vi "快捷菜单激活(表格).vi"(11 "菜单引用":refnum<k9>) -> ()   [LabVIEW 2021]
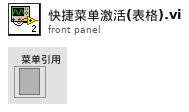
[diagram p1: front panel]
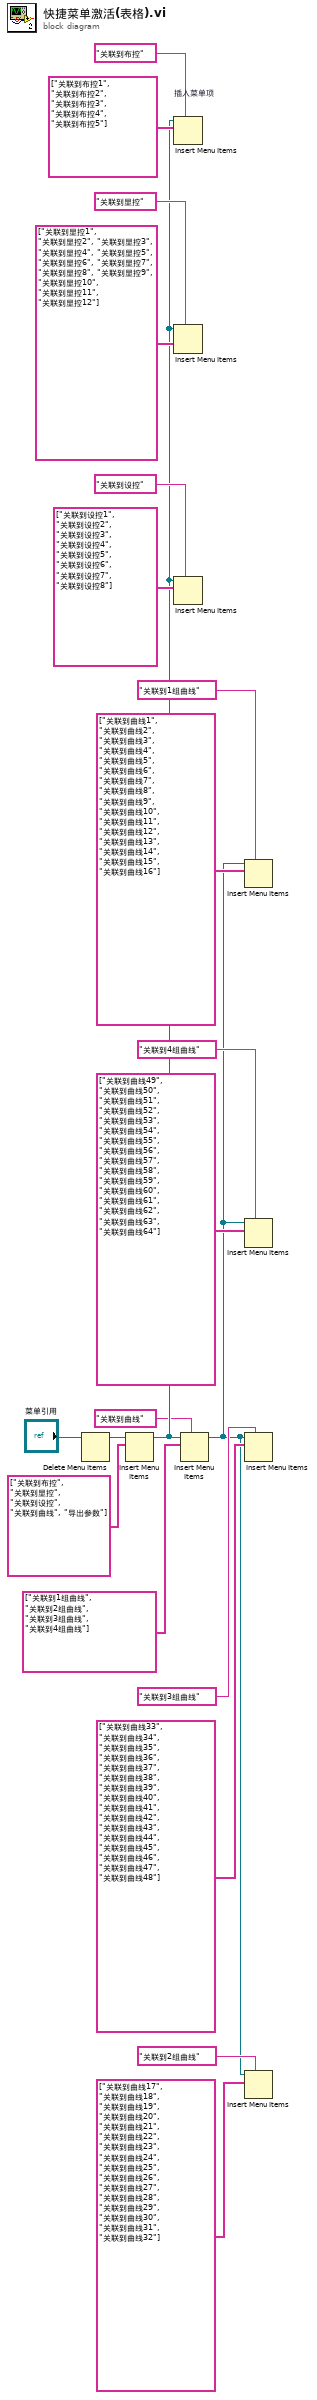
[diagram p0: block diagram]
diagram:
  n1 = Delete Menu Items(9:"菜单引用") -> (3:w21:refnum<k9>)  [unwired: 3 in, 1 out]
  n2 = Insert Menu Items ("插入菜单项")(8:string[] ["关联到布控", "关联到显控", "关联到设控", "关联到曲线", "导出参数"] ("项名称"), 9:w21) -> (3:w12:refnum<k9>)  [unwired: 4 in, 2 out]
  n3 = Insert Menu Items "插入菜单项"(5:"关联到布控" ("菜单标识符"), 8:string[] ["关联到布控1", "关联到布控2", "关联到布控3", "关联到布控4", "关联到布控5"] ("项名称"), 9:w12) -> ()  [unwired: 3 in, 3 out]
  n4 = Insert Menu Items ("插入菜单项")(5:"关联到显控" ("菜单标识符"), 7:string[] ["关联到显控1", "关联到显控2", "关联到显控3", "关联到显控4", "关联到显控5", "关联到显控6", "关联到显控7", "关联到显控8", "关联到显控9", "关联到显控10", "关联到显控11", "关联到显控12"] ("项标识符"), 9:w12) -> ()  [unwired: 3 in, 3 out]
  n5 = Insert Menu Items ("插入菜单项")(5:"关联到设控" ("菜单标识符"), 8:string[] ["关联到设控1", "关联到设控2", "关联到设控3", "关联到设控4", "关联到设控5", "关联到设控6", "关联到设控7", "关联到设控8"] ("项名称"), 9:w12) -> ()  [unwired: 3 in, 3 out]
  n6 = Insert Menu Items ("插入菜单项")(5:"关联到曲线" ("菜单标识符"), 8:string[] ["关联到1组曲线", "关联到2组曲线", "关联到3组曲线", "关联到4组曲线"] ("项名称"), 9:w12) -> (3:w1:refnum<k9>)  [unwired: 3 in, 2 out]
  n7 = Insert Menu Items ("插入菜单项")(5:"关联到1组曲线" ("菜单标识符"), 8:string[] ["关联到曲线1", "关联到曲线2", "关联到曲线3", "关联到曲线4", "关联到曲线5", "关联到曲线6", "关联到曲线7", "关联到曲线8", "关联到曲线9", "关联到曲线10", "关联到曲线11", "关联到曲线12", "关联到曲线13", "关联到曲线14", "关联到曲线15", "关联到曲线16"] ("项名称"), 9:w1) -> ()  [unwired: 3 in, 3 out]
  n8 = Insert Menu Items ("插入菜单项")(5:"关联到4组曲线" ("菜单标识符"), 8:string[] ["关联到曲线49", "关联到曲线50", "关联到曲线51", "关联到曲线52", "关联到曲线53", "关联到曲线54", "关联到曲线55", "关联到曲线56", "关联到曲线57", "关联到曲线58", "关联到曲线59", "关联到曲线60", "关联到曲线61", "关联到曲线62", "关联到曲线63", "关联到曲线64"] ("项名称"), 9:w1) -> ()  [unwired: 3 in, 3 out]
  n9 = Insert Menu Items ("插入菜单项")(5:"关联到3组曲线" ("菜单标识符"), 8:string[] ["关联到曲线33", "关联到曲线34", "关联到曲线35", "关联到曲线36", "关联到曲线37", "关联到曲线38", "关联到曲线39", "关联到曲线40", "关联到曲线41", "关联到曲线42", "关联到曲线43", "关联到曲线44", "关联到曲线45", "关联到曲线46", "关联到曲线47", "关联到曲线48"] ("项名称"), 9:w1) -> ()  [unwired: 3 in, 3 out]
  n10 = Insert Menu Items ("插入菜单项")(5:"关联到2组曲线" ("菜单标识符"), 8:string[] ["关联到曲线17", "关联到曲线18", "关联到曲线19", "关联到曲线20", "关联到曲线21", "关联到曲线22", "关联到曲线23", "关联到曲线24", "关联到曲线25", "关联到曲线26", "关联到曲线27", "关联到曲线28", "关联到曲线29", "关联到曲线30", "关联到曲线31", "关联到曲线32"] ("项名称"), 9:w1) -> ()  [unwired: 3 in, 3 out]
